vi "Test Serial Read.vi"() -> ()   [LabVIEW 2019, in "PGC2D.lvlib"]
uses:
  PGC2D.lvlib
  sandbox/Instrument.AML.GetAll--Cluster.ctl
panel:
  out "GetAll":T1
  out "error out":errorcluster
  in  "resource name":refnum<visa-resource-name>
  in  "error in (no error)":errorcluster
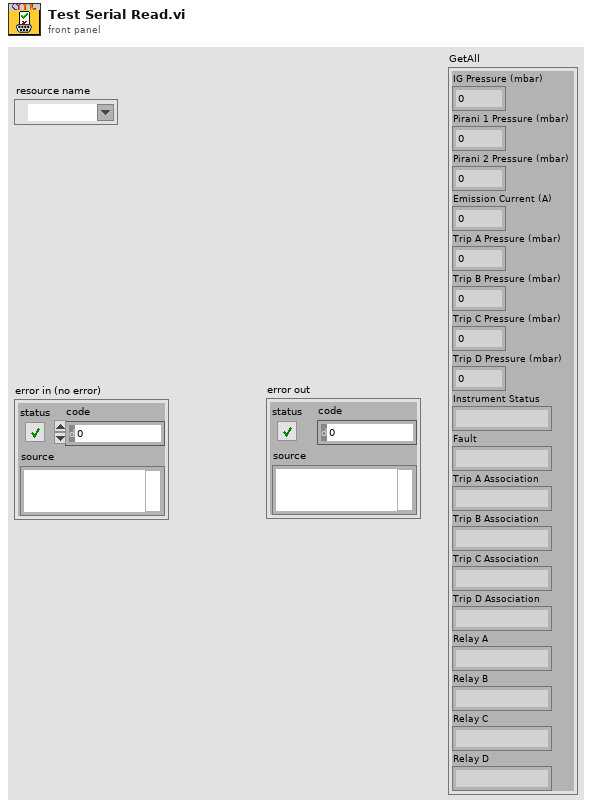
[diagram p1: front panel]
types:
  T1 = typedef "Instrument.AML.GetAll--Cluster.ctl" = cluster{"IG Pressure (mbar)":dbl, "Pirani 1 Pressure (mbar)":dbl, "Pirani 2 Pressure (mbar)":dbl, "Emission Current (A)":dbl, "Trip A Pressure (mbar)":dbl, "Trip B Pressure (mbar)":dbl, "Trip C Pressure (mbar)":dbl, "Trip D Pressure (mbar)":dbl, "Instrument Status":string, "Fault":string, "Trip A Association":string, "Trip B Association":string, "Trip C Association":string, "Trip D Association":string, "Relay A":string, "Relay B":string, "Relay C":string, "Relay D":string}
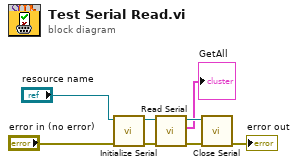
[diagram p0: block diagram]
diagram:
  n1 = call "Initialize Serial.vi"("error in (no error)"="error in (no error)", "VISA resource name"="resource name") -> ("error out"=w2:errorcluster, "VISA resource name out"=w7:refnum<visa-resource-name>)  [unwired: 8 in]
  n2 = call "Read Serial.vi"("error in (no error)"=w2, "VISA Reference"=w7) -> ("error out"=w3:errorcluster, "GetAll"=→"GetAll":T1, "VISA Reference out"=w6:refnum<visa-resource-name>)  [unwired: 7 in]
  n3 = call "Close Serial.vi"("error in (no error)"=w3, "VISA Reference"=w6) -> ("error out"=→"error out":errorcluster)  [unwired: 9 in]
